vi "5.Autocorrelation.vi"() -> ()   [LabVIEW 2018]
uses:
  <vilib>/Analysis/2dsp.llb/1D Auto Correlation (DBL).vi
  <vilib>/Analysis/NI_AALBase.lvlib
  <vilib>/measure/NI_MABase.lvlib
  <vilib>/Analysis/NI_AALPro.lvlib
panel:
  out "Waveform Graph 2":dbl[](graph)
  in  "Boolean":bool
  in  "nbr de signaux":dbl=2.0
  in  "stop":bool
  out "Waveform Graph":waveform(dbl)(graph)
  in  "Amplitude":dbl=1.0
  in  "Paramétre de siganl 2":T1={"Fréquence Echantioll"=1000.0, "nombre des echantionnage"=1000.0}
  in  "Paramétre de siganl":T2={"Amplitude"=1.0, "frequence"=2.0, "signal type"=enum."Sine Wave"}
  # "Bruit"
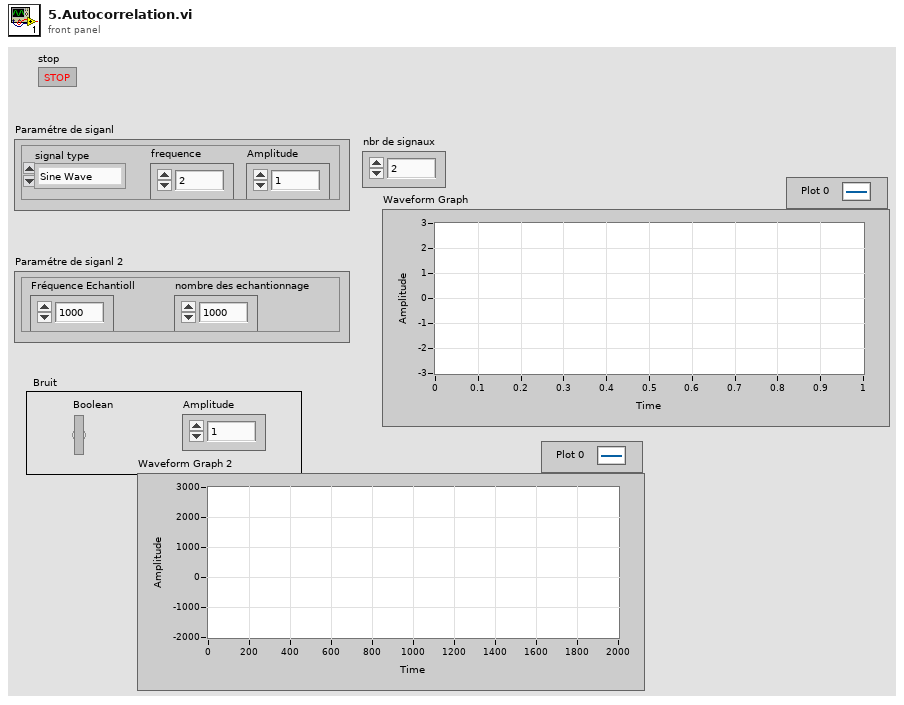
[diagram p1: front panel]
types:
  T1 = cluster{"Fréquence Echantioll":dbl, "nombre des echantionnage":dbl}
  T2 = cluster{"Amplitude":dbl, "frequence":dbl, "signal type":enum16{"Sine Wave", "Triangle Wave", "Square Wave", "Sawtooth Wave"}}
  T3 = enum16{"Sine Wave", "Triangle Wave", "Square Wave", "Sawtooth Wave"}
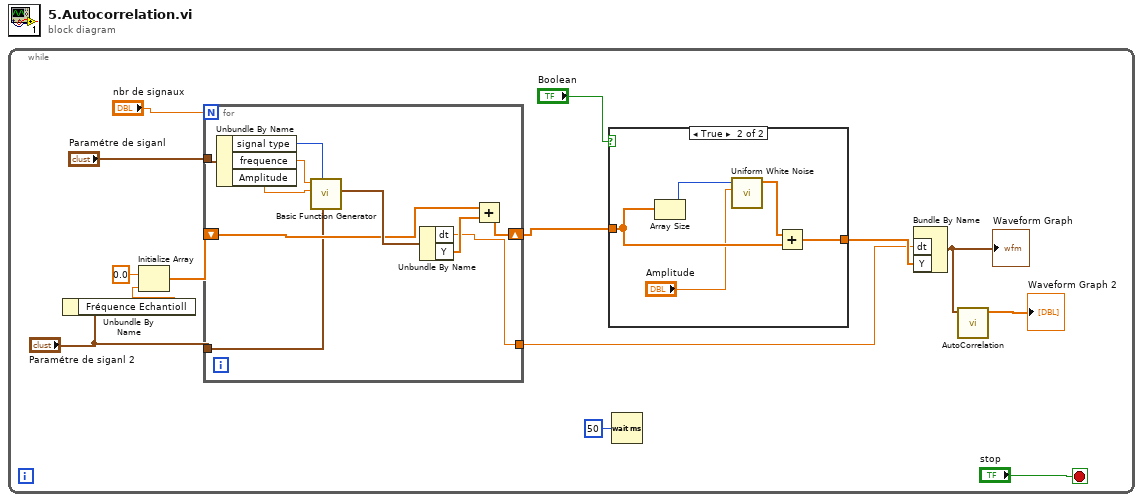
[diagram p0: block diagram]
diagram:
  n1 = while {
    stop <- "stop" stop-if-true
    n2 = Unbundle By Name("Paramétre de siganl 2") -> ("Fréquence Echantioll"=w12:dbl)
    n3 = Initialize Array(0.0 ("element"), w12) -> (w14:dbl[])
    n4 = for {
      N: "nbr de signaux" -> [_]
      shift-right: [w28] -> w10
      shift-left: w14 -> [w27]
      tunnel: "Paramétre de siganl 2" -> [w26]
      tunnel: [w25] -> w8
      tunnel: "Paramétre de siganl" -> [w21]
      n5 = Unbundle By Name(w21) -> ("signal type"=w24:T3, "frequence"=w23:dbl, "Amplitude"=w22:dbl)
      n6 = call <vilib>:"Basic Function Generator.vi"("sampling info"=w26, "signal type"=w24, "amplitude"=w22, "frequency"=w23) -> ("signal out"=w30:waveform(dbl))  [unwired: 5 in, 2 out]
      n7 = Unbundle By Name(w30) -> ("dt"=w25:dbl, "Y"=w29:dbl[])
      n8 = Add(x=w27, y=w29) -> (x+y=w28:dbl[])
    }
    n9 = case shown="True" "Boolean" {
      tunnel: w10 -> [w15 w18]
      tunnel: [w15 w16] -> w9
      frame False {
      }
      frame True {
        n10 = Array Size(array=w18) -> (size(s)=w20:i32)
        n11 = call <vilib>:"Uniform White Noise.vi"("amplitude"="Amplitude", "samples"=w20) -> ("uniform white noise"=w19:dbl[])  [unwired: 8 in, 1 out]
        n12 = Add(x=w19, y=w18) -> (x+y=w16:dbl[])
      }
    }
    n13 = Wait (ms)(milliseconds to wait=u32 50) -> ()  [unwired: 1 out]
    n14 = Bundle By Name("dt"=w8, "Y"=w9) -> (w2:waveform(dbl))  [unwired: 1 in]
    "Waveform Graph" <- w2
    n15 = call-poly <vilib>:"AutoCorrelation.vi"("X"=w2) -> ("Rxx"=→"Waveform Graph 2":dbl[])  [unwired: 9 in, 1 out]
  }
